vi "filterWheelClose.vi"   [LabVIEW 2017]
uses:
  globalDevices.vi
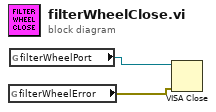
[diagram p0: block diagram]
diagram:
  n1 = global read "globalDevices.vi" "filterWheelError"() -> (w1:errorcluster)
  n2 = global read "globalDevices.vi" "filterWheelPort"() -> (w2:refnum<visa-resource-name>)
  n3 = VISA Close(VISA resource name=w2, error in (no error)=w1) -> ()  [unwired: 1 out]
